vi "getCursorProperties.vi"(8 "error in (no error)":errorcluster, 11 "QControl_Graph in":refnum<class "QControl_Graph.lvclass">) -> (0 "error out":errorcluster, 2 "Cursor Properties":T1={"Horizontal Line?"=TRUE, "Vertical Line?"=TRUE, "Timestamp"=enum."at BOTTOM", "time format (%H:%M:%S)"="%H:%M:%S", "size"=2, "font"={"Font Name"="Arial", "Size"=16, "Strikeout?"=FALSE, "Italic?"=FALSE, "Underline?"=FALSE, "Outline?"=FALSE, "Shadow"=FALSE, "Bold?"=FALSE}, "alignment(left, top)"={"Horizontal"=enum."center", "Vertical"=enum."center"}, "TextFormat"="%3$s\\n%2$.2f"} {"size" min=1 max=50}, 3 "QControl_Graph out":refnum<class "QControl_Graph.lvclass">)   [LabVIEW 2017, in "QControl_Graph.lvclass"]
uses:
  QControl_Graph.lvclass
  Font.ctl
  Alignment.Horizontal.ctl
  Alignment.Vertical.ctl
  Alignment.ctl
  Cursor Properties.ctl
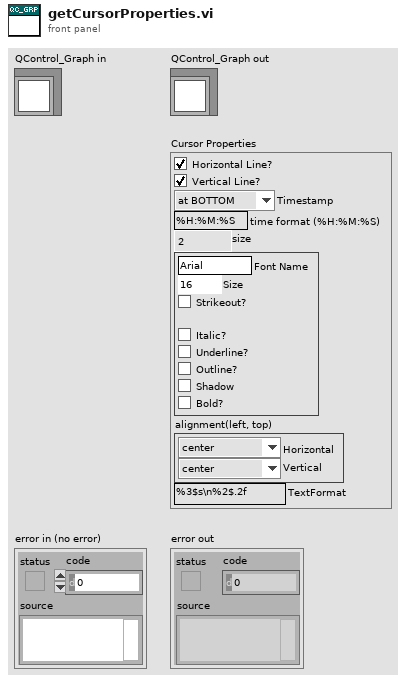
[diagram p1: front panel]
types:
  T1 = typedef "QControl_Graph.lvclass/Cursor Properties.ctl" = cluster{"Horizontal Line?":bool, "Vertical Line?":bool, "Timestamp":enum16{"at TOP", "at BOTTOM", "none"}, "time format (%H:%M:%S)":string, "size":i16, "font":T2, "alignment(left, top)":T3, "TextFormat":string}
  T2 = typedef "QControl_Graph.lvclass/Font.ctl" = cluster{"Font Name":string, "Size":i16, "Strikeout?":bool, "Italic?":bool, "Underline?":bool, "Outline?":bool, "Shadow":bool, "Bold?":bool}
  T3 = typedef "QControl_Graph.lvclass/Alignment.ctl" = cluster{"Horizontal":T4, "Vertical":T5}
  T4 = typedef "QControl_Graph.lvclass/Alignment.Horizontal.ctl" = enum16{"left", "center", "right"}
  T5 = typedef "QControl_Graph.lvclass/Alignment.Vertical.ctl" = enum16{"top", "center", "bottom"}
  T6 = typedef "QControl_Graph.lvclass/State Data.ctl" = cluster{"Data":bool, "Action Performed":refnum<user-event>, "Cursor Properties":T1}
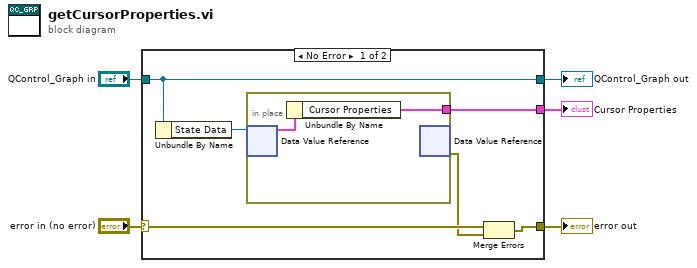
[diagram p0: block diagram]
diagram:
  n1 = case shown="No Error" "error in (no error)" {
    selector: "error in (no error)" -> [w11 w15]
    tunnel: [w7 w15] -> w3
    tunnel: [w10 w14] -> w4
    tunnel: "QControl_Graph in" -> [w10 w14]
    tunnel: [w8 _] -> w1
    frame No Error {
      n2 = Unbundle By Name(w10) -> ("State Data"=w9:refnum<data-value>)
      n3 = in-place {
        in-place-border: [w12] -> w8
        n4 = in-place-dvr #1(w9) -> (w13:T6)  [unwired: 1 out]
        n5 = Unbundle By Name(w13) -> ("Cursor Properties"=w12:T1)
        n6 = in-place-dvr #1() -> (w6:errorcluster)  [unwired: 1 in, 1 out]
      }
      n7 = Merge Errors(w11, w6) -> (w7:errorcluster)
    }
    frame Error {
    }
  }
  "error out" <- w3
  "QControl_Graph out" <- w4
  "Cursor Properties" <- w1
